vi "_convertExtensionArrayToString.vi"(8 "error in (no error)":errorcluster, 11 "Extensions":string[](array[string])) -> (0 "error out":errorcluster, 3 "Extension":string)   [LabVIEW 2020]
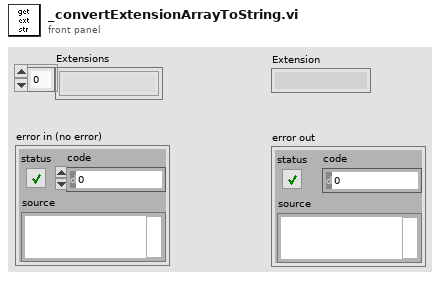
[diagram p1: front panel]
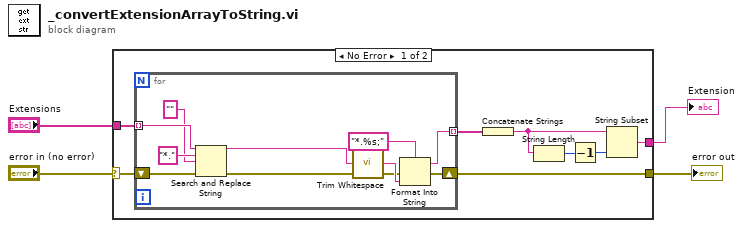
[diagram p0: block diagram]
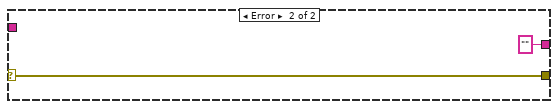
[diagram p2: hidden frame]
diagram:
  n1 = case shown="No Error" "error in (no error)" {
    selector: "error in (no error)" -> [w5 w23]
    tunnel: "Extensions" -> [w12 _]
    tunnel: [w7 ""] -> w3
    tunnel: [w6 w23] -> w2
    frame No Error {
      n2 = for {
        tunnel: w12 -> [w20] mode=indexing
        tunnel: [w21] -> w11 mode=indexing
        shift-right: [w17] -> w6
        shift-left: w5 -> [w15]
        n3 = Search and Replace String(input string=w20, search string="*.", replace string="" ("replace string (\"\")"), error in=w15) -> (result string=w13:string, error out=w14:errorcluster)  [unwired: 4 in, 2 out]
        n4 = call <vilib>:"Trim Whitespace.vi"("string"=w13) -> ("trimmed string"=w16:string)  [unwired: 1 in]
        n5 = Format Into String(format string="*.%s;", error in=w14, w16) -> (resulting string=w21:string, error out=w17:errorcluster)  [unwired: 1 in]
      }
      n6 = Concatenate Strings(w11) -> (w10:string)
      n7 = String Length(string=w10) -> (length=w9:i32)
      n8 = Decrement(x=w9) -> (x-1=w8:i32)
      n9 = String Subset(string=w10, length (rest)=w8) -> (substring=w7:string)  [unwired: 1 in]
    }
    frame Error {
    }
  }
  "Extension" <- w3
  "error out" <- w2
